vi "Get Description.vi"(8 "error in":errorcluster, 11 "data sharing framework custom device in":T1 format="%.0x") -> (0 "error out":errorcluster, 2 "description":string, 3 "data sharing framework custom deviceout":T1 format="%.0x")   [LabVIEW 2021, in "Data Sharing Framework Custom Device Scripting.lvlib"]
doc: "Reads the <b>description</b> field of the input Data Sharing Framework custom device."
uses:
  Data Sharing Framework Custom Device Scripting.lvlib
  <vilib>/NI VeriStand/Custom Device API/Custom Device Item Ref.ctl
  <vilib>/NI VeriStand/Custom Device API/Custom Device API.lvlib
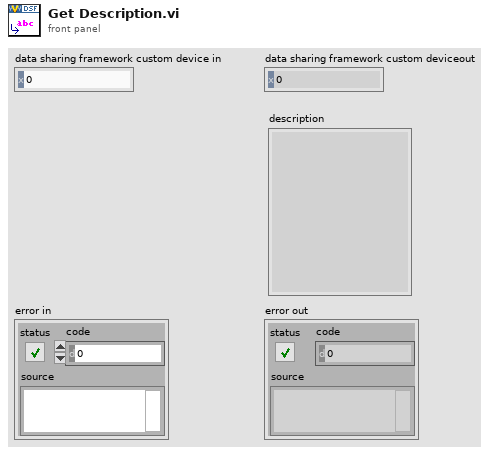
[diagram p1: front panel]
types:
  T1 = typedef "Custom Device API.lvlib/Custom Device Item Ref.ctl" = u64
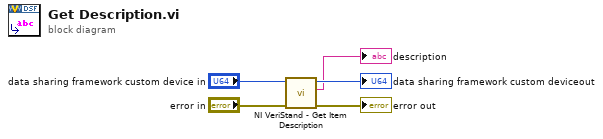
[diagram p0: block diagram]
diagram:
  n1 = call <vilib>:"NI VeriStand - Get Item Description.vi"("error in (no error)"="error in", "Item Ref in"="data sharing framework custom device in") -> ("error out"=→"error out":errorcluster, "Description"=→"description":string, "Item Ref out"=→"data sharing framework custom deviceout":T1)  [unwired: 6 in, 1 out]
